vi "InitiateServo.vi"(8 "error in":errorcluster, 10 "timeout_s":dbl=1.0, 11 "ServoSessionIn":u32) -> (0 "error out":errorcluster, 1 "Servo Failed":bool, 2 "Servo Done":bool, 3 "ServoSessionOut":u32, 5 "NumberAveragesCaptured":u16)   [LabVIEW 2016, in "Power Servo.lvlib"]
uses:
  Power Servo.lvlib
  <userlib>/_NI Power Servoing IP/HostRdl/NI Power Servoing IP New (Host).lvlib
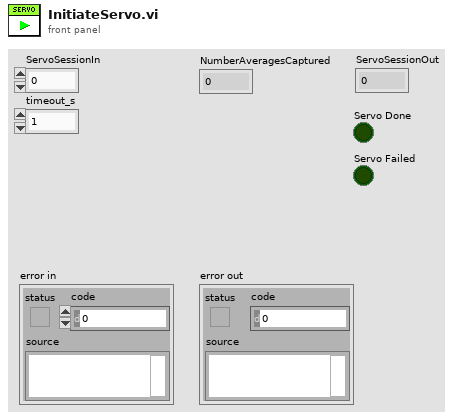
[diagram p1: front panel]
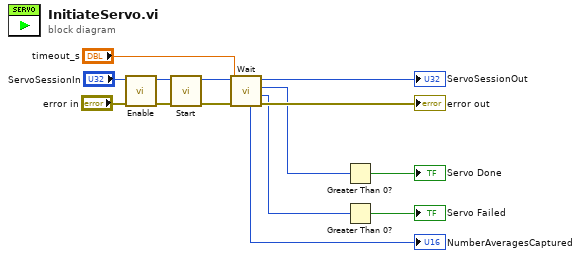
[diagram p0: block diagram]
diagram:
  n1 = call <userlib>:"Enable.vi"("error in"="error in", "SessionHandleIn"="ServoSessionIn") -> ("error out"=w1:errorcluster, "SessionHandleOut"=w3:u32)  [unwired: 8 in]
  n2 = call <userlib>:"Start.vi"("error in"=w1, "SessionHandleIn"=w3) -> ("error out"=w13:errorcluster, "SessionHandleOut"=w14:u32)  [unwired: 8 in]
  n3 = call <userlib>:"Wait.vi"("error in"=w13, "timeout"="timeout_s", "SessionHandleIn"=w14) -> ("error out"=→"error out":errorcluster, "Failed"=w8:u16, "Done"=w6:u16, "SessionHandleOut"=→"ServoSessionOut":u32, "NumberAveragesCaptured"=→"NumberAveragesCaptured":u16)  [unwired: 4 in]
  n4 = Greater Than 0?(x=w6) -> (x > 0?=→"Servo Done":bool)
  n5 = Greater Than 0?(x=w8) -> (x > 0?=→"Servo Failed":bool)
